vi "SGDA-Close Hardware.vi"(4 "error in (no error)":errorcluster, 7 "Stop PXI Server (T)":bool=TRUE) -> (0 "error out":errorcluster)   [LabVIEW 2020]
doc: "Sends <B>Start</B> notifier to DAQ thread to begin measurement."
uses:
  SGDA-Globals.vi
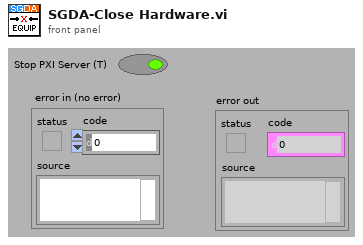
[diagram p1: front panel]
types:
  T1 = typedef "Hardware Destination.ctl" = enum16{"None", "PXI", "TDT", "NI", "TDTSIM"}
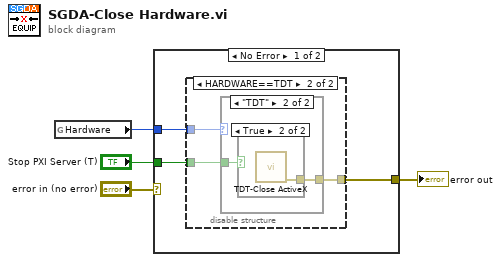
[diagram p0: block diagram]
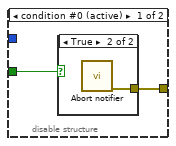
[diagram p2: hidden frame]
diagram:
  n1 = global read "SGDA-Globals.vi" "Hardware"() -> (w3:T1)
  n2 = case shown="No Error" "error in (no error)" {
    selector: "error in (no error)" -> [_ w17]
    tunnel: w3 -> [w7 _]
    tunnel: [w6 w17] -> w2
    tunnel: "Stop PXI Server (T)" -> [w5 _]
    frame No Error {
      n3 = disable-structure shown="HARDWARE==TDT" {
        disable-tunnel: w7 -> [_ w12]
        disable-tunnel: [w9 w13] -> w6
        disable-tunnel: w5 -> [w8 w11]
        frame condition #0 (active) {
          n4 = case shown="True" w8 {
            tunnel: [_ w10] -> w9
            frame False {
            }
            frame True {
              n5 = call "Abort notifier.vi"() -> ("error out"=w10:errorcluster)  [unwired: 6 in, 1 out]
            }
          }
        }
        frame condition #1 {
          n6 = case shown="\"TDT\"" w12 {
            tunnel: [_ w15] -> w13
            tunnel: w11 -> [_ w14]
            frame "None", Default {
            }
            frame "TDT" {
              n7 = case shown="True" w14 {
                tunnel: [_ w16] -> w15
                frame False {
                }
                frame True {
                  n8 = call "TDT-Close ActiveX.vi"() -> ("error out"=w16:errorcluster)  [unwired: 15 in]
                }
              }
            }
          }
        }
      }
    }
    frame Error {
    }
  }
  "error out" <- w2
